vi "Protocol.Convert Data to DTC Frame.vi"(11 "Data":dbl[](array[numeric])) -> (3 "DTC Frame":u8[](array[numeric]) format="%.0b")   [LabVIEW 2019, in "J1939 Addon Engine.lvlib"]
uses:
  J1939 Addon Engine.lvlib
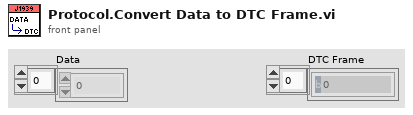
[diagram p1: front panel]
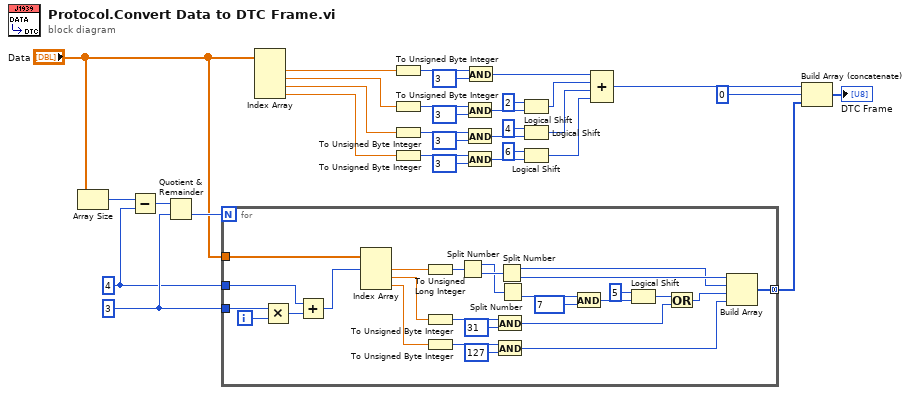
[diagram p0: block diagram]
diagram:
  w4 = 3 ("x")
  w3 = 4 ("x")
  n1 = Array Size(array="Data") -> (size(s)=w7:i32)
  n2 = Subtract(x=w7, y=w3) -> (x-y=w8:i32)
  n3 = Quotient & Remainder(x=w8, y=w4) -> (floor(x/y)=w5:i32)  [unwired: 1 out]
  n4 = for {
    N: w5 -> [_]
    tunnel: "Data" -> [w46]
    tunnel: [w38] -> w6 mode=concatenating
    tunnel: w4 -> [w36]
    tunnel: w3 -> [w34]
    i -> [w37]
    n5 = Multiply(x=w36, y=w37) -> (x*y=w35:i32)
    n6 = Add(x=w34, y=w35) -> (x+y=w33:i32)
    n7 = Index Array(array=w46, index #1=w33) -> (element #1=w45:dbl, element #2=w44:dbl, element #3=w43:dbl)  [unwired: 2 in]
    n8 = To Unsigned Long Integer(number=w45) -> (unsigned 32bit integer=w59:u32)
    n9 = To Unsigned Byte Integer(number=w44) -> (unsigned 8bit integer=w51:u8)
    n10 = To Unsigned Byte Integer(number=w43) -> (unsigned 8bit integer=w53:u8)
    n11 = Split Number(x=w59) -> (hi(x)=w57:u16, lo(x)=w58:u16)
    n12 = And(x=w51, y=u8 31) -> (x .and. y?=w47:u8)
    n13 = And(x=w53, y=u8 127) -> (x .and. y?=w39:u8)
    n14 = Split Number(x=w58) -> (hi(x)=w41:u8, lo(x)=w42:u8)
    n15 = Split Number(x=w57) -> (lo(x)=w55:u8)  [unwired: 1 out]
    n16 = And(x=w55, y=u8 7) -> (x .and. y?=w50:u8)
    n17 = Logical Shift(y=i16 5, x=w50) -> (x << y=w48:u8)
    n18 = Or(x=w48, y=w47) -> (x .or. y?=w40:u8)
    n19 = Build Array(w42, w41, w40, w39) -> (w38:u8[])
  }
  n20 = Index Array(array="Data") -> (element #1=w32:dbl, element #2=w23:dbl, element #3=w22:dbl, element #4=w21:dbl)  [unwired: 4 in]
  n21 = To Unsigned Byte Integer(number=w32) -> (unsigned 8bit integer=w31:u8)
  n22 = To Unsigned Byte Integer(number=w23) -> (unsigned 8bit integer=w28:u8)
  n23 = To Unsigned Byte Integer(number=w22) -> (unsigned 8bit integer=w27:u8)
  n24 = To Unsigned Byte Integer(number=w21) -> (unsigned 8bit integer=w24:u8)
  n25 = And(x=w28, y=u8 3) -> (x .and. y?=w19:u8)
  n26 = And(x=w27, y=u8 3) -> (x .and. y?=w18:u8)
  n27 = And(x=w24, y=u8 3) -> (x .and. y?=w20:u8)
  n28 = And(x=w31, y=u8 3) -> (x .and. y?=w14:u8)
  n29 = Logical Shift(y=i16 2, x=w19) -> (x << y=w13:u8)
  n30 = Logical Shift(y=i16 4, x=w18) -> (x << y=w12:u8)
  n31 = Logical Shift(y=i16 6, x=w20) -> (x << y=w11:u8)
  n32 = Compound Arithmetic op=ADD(w14, w13, w12, w11) -> (w10:u8)
  n33 = Build Array (concatenate)(w10, u8 0 ("element"), w6) -> (→"DTC Frame":u8[])
